vi "LogTracePoint.vi"(8 "error in (no error)":errorcluster, 9 "log string":string, 10 "tracepoint name":string, 11 "service in":refnum<class "IcmMessageService.lvclass">) -> (0 "error out":errorcluster, 3 "service out":refnum<class "IcmMessageService.lvclass">)   [LabVIEW 2017, in "IcmMessageService.lvclass"]
doc: "Writes an instance of a tracepoint to a temporary tracelog file on the device disk and sends the instance to NI InsightCM Server to be saved in its tracelog. If the tracepoint is disabled, this VI ignores the input."
uses:
  <vilib>/addons/InsightCM/MessageBus/MessageService/IcmMessageService.lvclass
  <vilib>/addons/InsightCM/MessageBus/MessageService/IcmMessageService.lvclass/IcmMessageService.ctl
  C:/Program Files (x86)/National Instruments/LabVIEW 2017/vi.lib/addons/InsightCM/Binaries/LabviewMessageAdapter.dll
  Binaries/LabviewMessageAdapter.dll
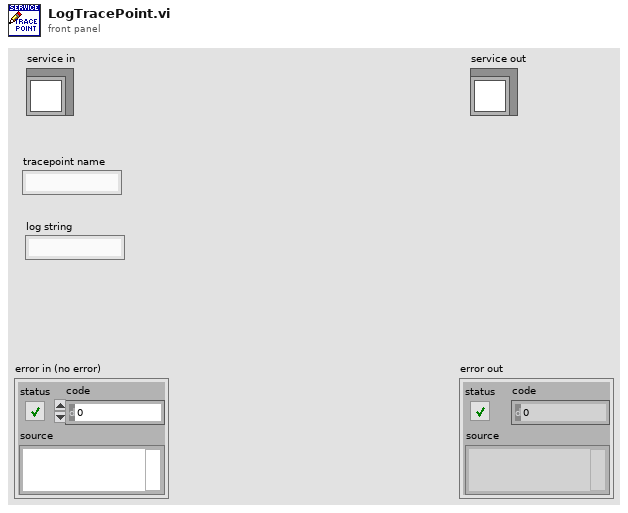
[diagram p1: front panel]
types:
  T1 = typedef "MessageServiceDvr.ctl" = refnum<data-value>
  T2 = typedef "MessageServiceData.ctl" = cluster{"Service":refnum<k24>}
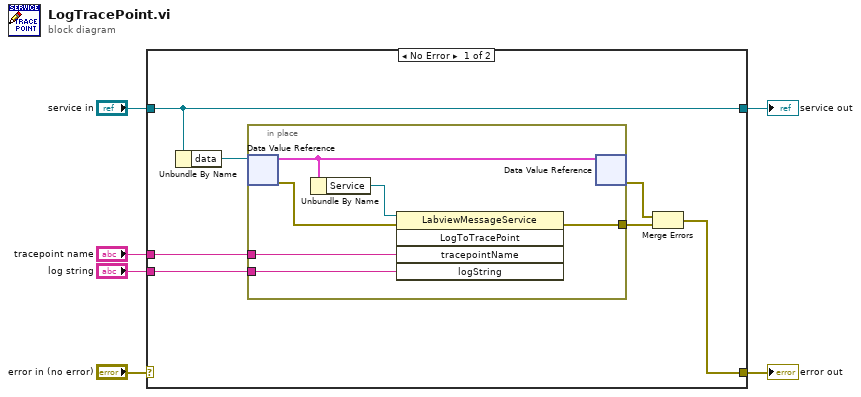
[diagram p0: block diagram]
diagram:
  n1 = case shown="No Error" "error in (no error)" {
    selector: "error in (no error)" -> [_ w21]
    tunnel: [w9 w21] -> w5
    tunnel: [w13 w20] -> w3
    tunnel: "service in" -> [w13 w20]
    tunnel: "tracepoint name" -> [w8 _]
    tunnel: "log string" -> [w7 _]
    frame No Error {
      n2 = Unbundle By Name(w13) -> ("data"=w12:T1)
      n3 = in-place {
        in-place-border: [w16] -> w10
        in-place-border: w8 -> [w15]
        in-place-border: w7 -> [w14]
        n4 = in-place-dvr #1(w12) -> (w19:T2, w17:errorcluster)
        n5 = Unbundle By Name(w19) -> ("Service"=w18:refnum<k24>)
        n6 = invoke class="LabviewMessageService" method="LogToTracePoint"(reference=w18, error in=w17, "tracepointName"=w15, "logString"=w14) -> (error out=w16:errorcluster)  [unwired: 1 in, 4 out]
        n7 = in-place-dvr #1(w19) -> (w11:errorcluster)  [unwired: 1 out]
      }
      n8 = Merge Errors(w11, w10) -> (w9:errorcluster)
    }
    frame Error {
    }
  }
  "error out" <- w5
  "service out" <- w3
